vi "udp_client_test.vi"() -> ()   [LabVIEW 2018]
panel:
  out "sz":i32
  out "data":string
  out "Array":dbl[](array[numeric])=[1.0, 2.0, 3.0, 4.0, 5.0, 6.0]
  in  "Init Array":dbl[](array[numeric])=[1.0, 2.0, 3.0, 4.0, 5.0, 6.0]
  in  "listening port":u16=50005
  in  "IP address":string="172.22.11.2"
  in  "server port":u16=60006
  out "stop":bool
  # "UDP client test (transmit)"
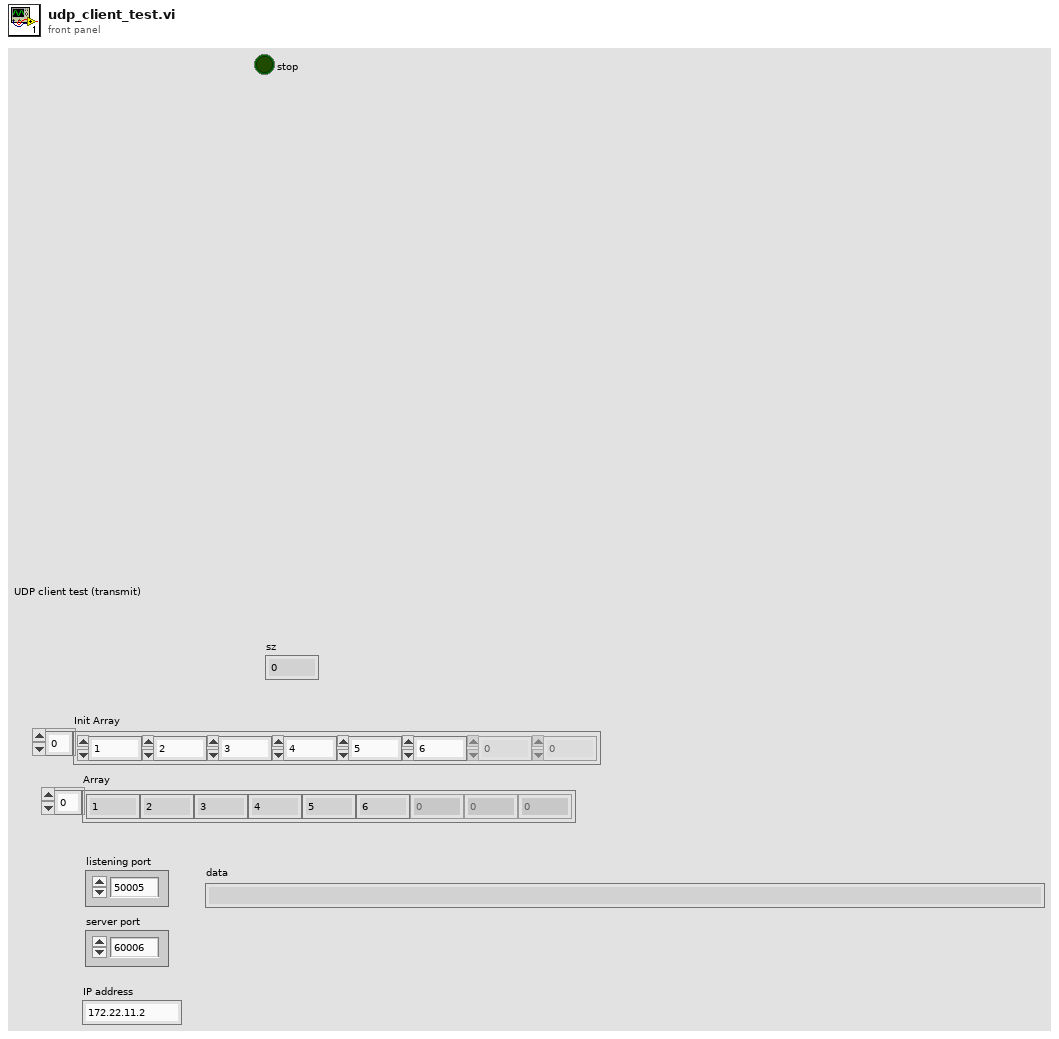
[diagram p1: front panel]
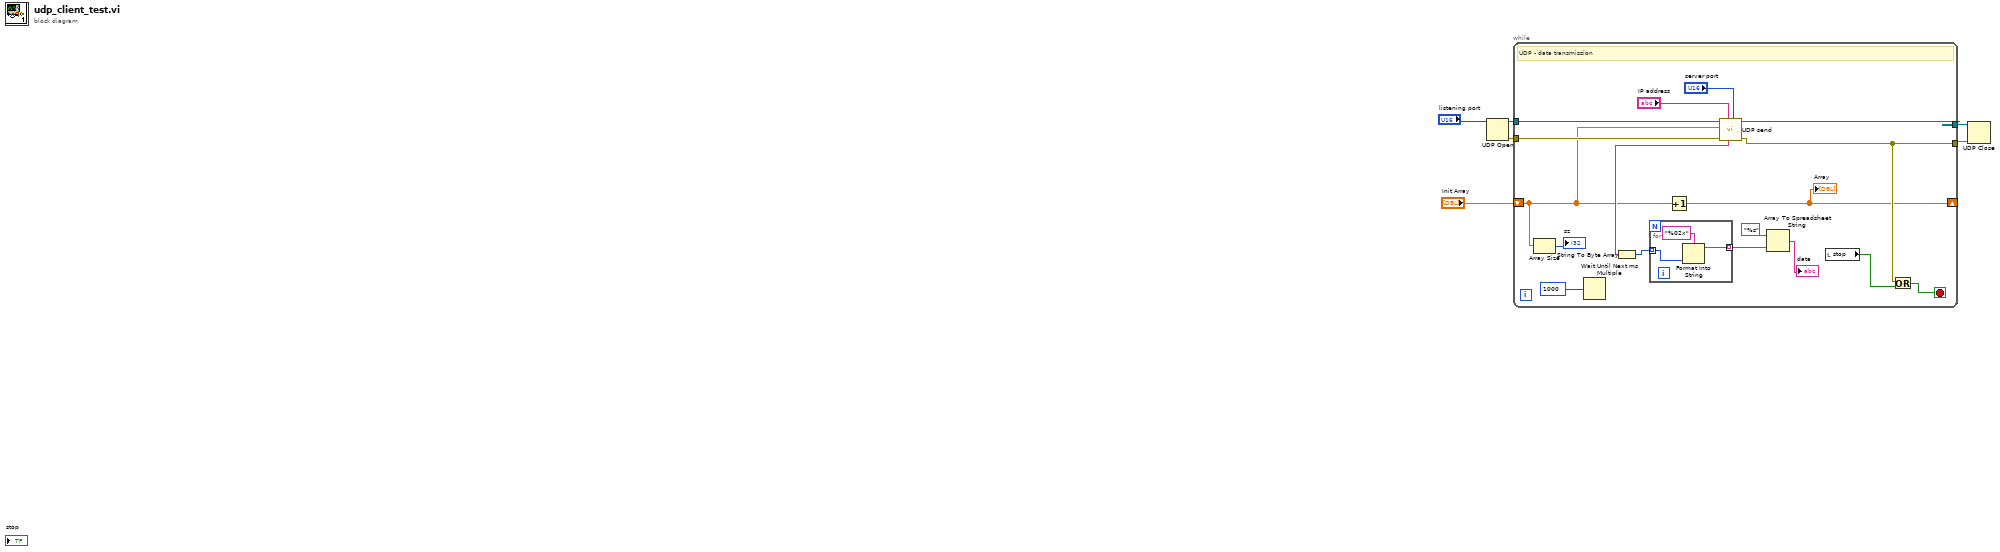
[diagram p0: block diagram]
diagram:
  n1 = UDP Open(11:"listening port") -> (port=w6:refnum<k16>, 0:w5:errorcluster)  [unwired: 4 in, 1 out]
  n2 = while {
    tunnel: w6 -> [w23]
    tunnel: w5 -> [w22]
    tunnel: [w21] -> w4
    tunnel: [w17] -> w3
    shift-right: [w7] -> _
    shift-left: "Init Array" -> [w8]
    stop <- w18 stop-if-true
    # "UDP - data transmission"
    n3 = Array Size(array=w8) -> (size(s)=→"sz":i32)
    n4 = Wait Until Next ms Multiple(millisecond multiple=1000) -> ()  [unwired: 1 out]
    n5 = Increment(x=w8) -> (x+1=w7:dbl[])
    "Array" <- w7
    n6 = call "UDP send.vi"("port or service name"="server port", "IP address"="IP address", "error in"=w22, "Array"=w8, "connection ID in"=w23) -> ("error out"=w17:errorcluster, "connection ID out"=w21:refnum<k16>, "raw data"=w12:string)  [unwired: 4 in]
    n7 = String To Byte Array(string=w12) -> (unsigned byte array=w11:u8[])
    n8 = for {
      tunnel: [w26] -> w10 mode=indexing
      tunnel: w11 -> [w24] mode=indexing
      n9 = Format Into String(format string="%02x", w24) -> (resulting string=w26:string)  [unwired: 2 in, 1 out]
    }
    n10 = Array To Spreadsheet String(array=w10, 3:"%s") -> (spreadsheet string=→"data":string)  [unwired: 1 in]
    n11 = local read "stop"() -> (w16:bool)
    n12 = Or(x=w17, y=w16) -> (x .or. y?=w18:bool)
  }
  n13 = UDP Close(connection ID=w4, 8:w3) -> ()  [unwired: 2 out]
